vi "_Get Server Ref.vi"(7 "IsSimplicityServer":bool) -> (0 "error out":errorcluster, 2 "Locked":bool, 3 "Server Ref":T1)   [LabVIEW 2012]
uses:
  Type/_Server Reference.ctl
  <vilib>/registry/registry.llb/Registry SAM.ctl
  <vilib>/registry/registry.llb/Read Registry Value Simple STR.vi
panel:
  # "It takes normally 25-30 ms to complete"
  # "To be called once at the start of each DLL function.\nThe DLL function must close the Application Reference before exiting."
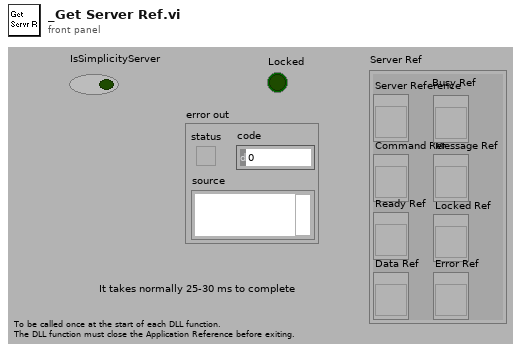
[diagram p1: front panel]
types:
  T1 = typedef "_Server Reference.ctl" = cluster{"Server Reference":refnum<vi>, "Command Ref":refnum<vi>, "Message Ref":refnum<vi>, "Ready Ref":refnum<vi>, "Locked Ref":refnum<vi>, "Data Ref":refnum<vi>, "Error Ref":refnum<vi>, "Busy Ref":refnum<vi>}
  T2 = typedef "Registry SAM.ctl" = enum32{"KEY_QUERY_VALUE", "KEY_SET_VALUE", "KEY_CREATE_SUB_KEY", "KEY_ENUMERATE_SUB_KEYS", "KEY_NOTIFY", "KEY_CREATE_LINK", "KEY_READ", "KEY_WRITE", "KEY_ALL_ACCESS", "KEY_READ | KEY_WRITE"}
  T3 = typedef "Registry refnum.ctl" = refnum<k1>
  T4 = cluster{"Server Reference":refnum<vi>, "Ctl Refnum":refnum<vi>, "Ctl Refnum":refnum<vi>, "Ctl Refnum":refnum<vi>, "Ctl Refnum":refnum<vi>, "Ctl Refnum":refnum<vi>, "Ctl Refnum":refnum<vi>, "Ctl Refnum":refnum<vi>}
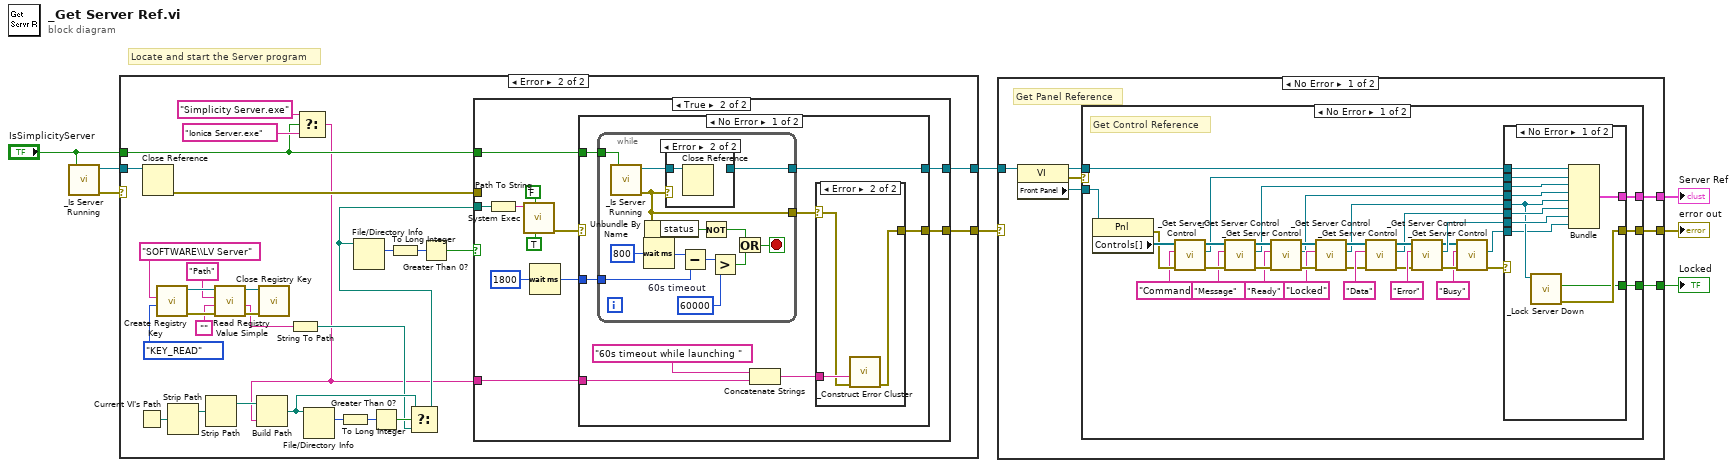
[diagram p0: block diagram]
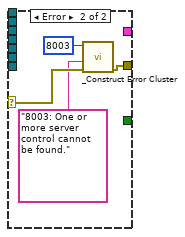
[diagram p2: hidden frame]
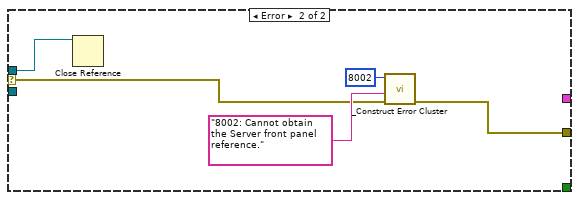
[diagram p3: hidden frame]
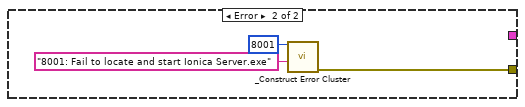
[diagram p4: hidden frame]
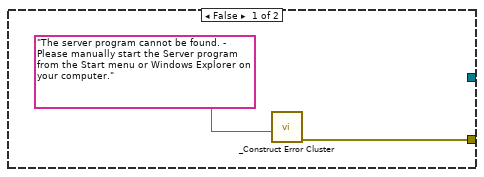
[diagram p6: hidden frame]
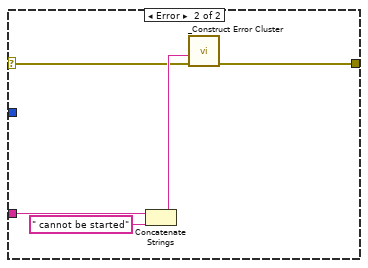
[diagram p9: hidden frame]
diagram:
  # "Locate and start the Server program"
  n1 = call "_Is Server Running.vi"("IsSimplicityServer"="IsSimplicityServer") -> ("error out"=w7:errorcluster, "Server Reference"=w8:refnum<vi>)  [unwired: 1 in, 4 out]
  n2 = case shown="Error" w7 {
    tunnel: w8 -> [w9 w25]
    tunnel: [w9 w24] -> w6
    tunnel: [_ w23] -> w5
    tunnel: "IsSimplicityServer" -> [_ w11]
    frame No Error {
      # "The Server is already running"
    }
    frame Error {
      n3 = Current VI's Path() -> (path=w29:path)
      n4 = Close Reference(reference=w25) -> (error out=w22:errorcluster)  [unwired: 1 in]
      n5 = call <vilib>:"Create Registry Key.vi"("security access mask (KEY_READ | KEY_WRITE)"=Registry_SAM."KEY_READ", "subkey"="SOFTWARE\\LV Server") -> ("error out"=w35:errorcluster, "refnum out"=w36:T3)  [unwired: 2 in, 6 out]
      n6 = Strip Path(path=w29) -> (stripped path=w28:path)  [unwired: 1 out]
      n7 = Strip Path(path=w28) -> (stripped path=w27:path)  [unwired: 1 out]
      n8 = call-poly <vilib>:"Read Registry Value Simple.vi"("error in (no error)"=w35, "default data"="", "value"="Path", "refnum"=w36) -> ("error out"=w34:errorcluster, "String/Binary data"=w30:string, "refnum out"=w33:T3)  [unwired: 3 out]
      n9 = call <vilib>:"Close Registry Key.vi"("error in (no error)"=w34, "refnum"=w33) -> ()  [unwired: 6 out]
      n10 = String To Path(string=w30) -> (path=w18:path)
      n11 = Select(t="Simplicity Server.exe", s=w11, f="Ionica Server.exe") -> (s? t:f=w10:string)
      n12 = Build Path(base path=w27, name or relative path=w10) -> (appended path=w19:path)
      n13 = File/Directory Info(path=w19) -> (size=w21:i64)  [unwired: 1 in, 6 out]
      n14 = To Long Integer(number=w21) -> (32bit integer=w26:i32)
      n15 = Greater Than 0?(x=w26) -> (x > 0?=w20:bool)
      n16 = Select(t=w19, s=w20, f=w18) -> (s? t:f=w14:path)
      n17 = File/Directory Info(path=w14) -> (size=w17:i64)  [unwired: 1 in, 6 out]
      n18 = To Long Integer(number=w17) -> (32bit integer=w16:i32)
      n19 = Greater Than 0?(x=w16) -> (x > 0?=w15:bool)
      n20 = case shown="True" w15 {
        tunnel: w14 -> [_ w51]
        tunnel: [w40 w43] -> w23
        tunnel: w22 -> [_ _]
        tunnel: [_ w45] -> w24
        tunnel: w10 -> [_ w42]
        tunnel: w11 -> [_ w41]
        frame False {
          n21 = call "_Construct Error Cluster.vi"("reason"="The server program cannot be found. - Please manually start the Server program from the Start menu or Windows Explorer on your computer.") -> ("error out"=w40:errorcluster)  [unwired: 3 in, 3 out]
        }
        frame True {
          n22 = Path To String(path=w51) -> (string=w50:string)
          n23 = call <vilib>:"System Exec.vi"("run minimized? (F)"=TRUE, "wait until completion? (T)"=FALSE, "command line"=w50) -> ("error out"=w44:errorcluster)  [unwired: 3 in, 5 out]
          n24 = Wait (ms)(milliseconds to wait=u32 1800) -> (millisecond timer value=w46:u32)
          n25 = case shown="No Error" w44 {
            selector: w44 -> [_ w79]
            tunnel: w46 -> [w59 _]
            tunnel: [w58 _] -> w45
            tunnel: [w54 w78] -> w43
            tunnel: w42 -> [w57 w82]
            tunnel: w41 -> [w52 _]
            frame No Error {
              n26 = while {
                tunnel: w59 -> [w73]
                tunnel: [w68] -> w58
                tunnel: [w64] -> w53
                tunnel: w52 -> [w63]
                stop <- w70 stop-if-true
                w71 = u32 60000  # 60s timeout
                n27 = call "_Is Server Running.vi"("IsSimplicityServer"=w63) -> ("error out"=w64:errorcluster, "Server Reference"=w69:refnum<vi>)  [unwired: 1 in, 4 out]
                n28 = Wait (ms)(milliseconds to wait=u32 800) -> (millisecond timer value=w74:u32)
                n29 = Unbundle By Name(w64) -> ("status"=w66:bool)
                n30 = case shown="Error" w64 {
                  tunnel: w69 -> [w76 w77]
                  tunnel: [w76 _] -> w68
                  frame No Error {
                  }
                  frame Error {
                    n31 = Close Reference(reference=w77) -> ()  [unwired: 1 in, 1 out]
                  }
                }
                n32 = Subtract(x=w74, y=w73) -> (x-y=w72:u32)
                n33 = Not(x=w66) -> (.not. x?=w65:bool)
                n34 = Greater?(x=w72, y=w71) -> (0:w67:bool)
                n35 = Or(x=w65, y=w67) -> (x .or. y?=w70:bool)
              }
              n36 = Concatenate Strings("60s timeout while launching " ("f"), w57) -> (w55:string)
              n37 = case shown="Error" w53 {
                selector: w53 -> [_ w60]
                tunnel: w55 -> [_ w62]
                tunnel: [_ w61] -> w54
                frame No Error {
                }
                frame Error {
                  n38 = call "_Construct Error Cluster.vi"("error in"=w60, "reason"=w62) -> ("error out"=w61:errorcluster)  [unwired: 2 in, 3 out]
                }
              }
            }
            frame Error {
              n39 = Concatenate Strings(w82, " cannot be started" ("f")) -> (w80:string)
              n40 = call "_Construct Error Cluster.vi"("error in"=w79, "reason"=w80) -> ("error out"=w78:errorcluster)  [unwired: 2 in, 3 out]
            }
          }
        }
      }
    }
  }
  n41 = case shown="No Error" w5 {
    tunnel: w6 -> [w89 _]
    tunnel: [w88 w146] -> w4
    tunnel: [w84 _] -> w3
    tunnel: [w83 _] -> w2
    frame No Error {
      # "Get Panel Reference"
      n42 = property class="VI"(reference=w89) -> (reference out=w85:refnum<vi>, error out=w86:errorcluster, "Front Panel"=w87:refnum<vi>)  [unwired: 1 in]
      n43 = case shown="No Error" w86 {
        selector: w86 -> [_ w141]
        tunnel: w87 -> [w123 _]
        tunnel: [w104 w143] -> w88
        tunnel: w85 -> [w103 w140]
        tunnel: [w96 _] -> w84
        tunnel: [w95 _] -> w83
        frame No Error {
          # "Get Control Reference"
          n44 = property class="Pnl"(reference=w123) -> (error out=w121:errorcluster, "Controls[]"=w122:refnum<vi>[])  [unwired: 1 in, 1 out]
          n45 = call "_Get Server Control.vi"("error in (no error)"=w121, "Control Name"="Command", "All Controls[]"=w122) -> ("error out"=w119:errorcluster, "Ctl Refnum"=w102:refnum<vi>, "All Controls[] out"=w118:refnum<vi>[])  [unwired: 2 out]
          n46 = call "_Get Server Control.vi"("error in (no error)"=w119, "Control Name"="Message", "All Controls[]"=w118) -> ("error out"=w116:errorcluster, "Ctl Refnum"=w101:refnum<vi>, "All Controls[] out"=w115:refnum<vi>[])  [unwired: 2 out]
          n47 = call "_Get Server Control.vi"("error in (no error)"=w116, "Control Name"="Ready", "All Controls[]"=w115) -> ("error out"=w111:errorcluster, "Ctl Refnum"=w100:refnum<vi>, "All Controls[] out"=w110:refnum<vi>[])  [unwired: 2 out]
          n48 = call "_Get Server Control.vi"("error in (no error)"=w111, "Control Name"="Locked", "All Controls[]"=w110) -> ("error out"=w106:errorcluster, "Ctl Refnum"=w99:refnum<vi>, "All Controls[] out"=w112:refnum<vi>[])  [unwired: 2 out]
          n49 = call "_Get Server Control.vi"("error in (no error)"=w106, "Control Name"="Data", "All Controls[]"=w112) -> ("error out"=w105:errorcluster, "Ctl Refnum"=w98:refnum<vi>, "All Controls[] out"=w113:refnum<vi>[])  [unwired: 2 out]
          n50 = call "_Get Server Control.vi"("error in (no error)"=w105, "Control Name"="Error", "All Controls[]"=w113) -> ("error out"=w92:errorcluster, "Ctl Refnum"=w97:refnum<vi>, "All Controls[] out"=w93:refnum<vi>[])  [unwired: 2 out]
          n51 = call "_Get Server Control.vi"("error in (no error)"=w92, "Control Name"="Busy", "All Controls[]"=w93) -> ("error out"=w94:errorcluster, "Ctl Refnum"=w90:refnum<vi>)  [unwired: 3 out]
          n52 = case shown="No Error" w94 {
            selector: w94 -> [_ w138]
            tunnel: [w126 w136] -> w104
            tunnel: w103 -> [w134 _]
            tunnel: w102 -> [w133 _]
            tunnel: w101 -> [w132 _]
            tunnel: w100 -> [w131 _]
            tunnel: w99 -> [w127 _]
            tunnel: w98 -> [w130 _]
            tunnel: w97 -> [w129 _]
            tunnel: [w128 _] -> w96
            tunnel: [w125 _] -> w95
            tunnel: w90 -> [w124 _]
            frame No Error {
              n53 = call "_Lock Server Down.vi"("Locked Ref"=w127) -> ("error out"=w126:errorcluster, "Locked"=w125:bool)  [unwired: 1 in, 4 out]
              n54 = Bundle("Server Reference"=w134, "Ctl Refnum"=w133, "Ctl Refnum"=w132, "Ctl Refnum"=w131, "Ctl Refnum"=w127, "Ctl Refnum"=w130, "Ctl Refnum"=w129, "Ctl Refnum"=w124) -> (w128:T4)  [unwired: 1 out]
            }
            frame Error {
              n55 = call "_Construct Error Cluster.vi"("error in"=w138, "reason"="8003: One or more server control cannot be found.", "errorCode"=8003) -> ("error out"=w136:errorcluster)  [unwired: 1 in, 3 out]
            }
          }
        }
        frame Error {
          n56 = Close Reference(reference=w140) -> ()  [unwired: 1 in, 1 out]
          n57 = call "_Construct Error Cluster.vi"("error in"=w141, "reason"="8002: Cannot obtain the Server front panel reference.", "errorCode"=8002) -> ("error out"=w143:errorcluster)  [unwired: 1 in, 3 out]
        }
      }
    }
    frame Error {
      n58 = call "_Construct Error Cluster.vi"("reason"="8001: Fail to locate and start Ionica Server.exe", "errorCode"=8001) -> ("error out"=w146:errorcluster)  [unwired: 2 in, 3 out]
    }
  }
  "error out" <- w4
  "Server Ref" <- w3
  "Locked" <- w2
